vi "LCD Retarder (No Objects).vi"(8 "error in":errorcluster) -> (0 "errorOUT":errorcluster, 3 "LCD out":T1)   [LabVIEW 2015]
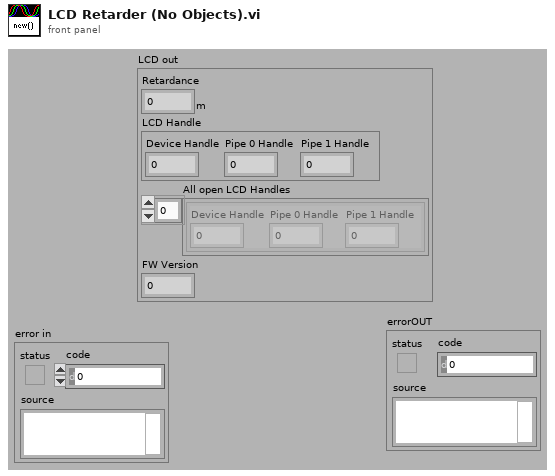
[diagram p1: front panel]
types:
  T1 = cluster{"Retardance":dbl[unit], "LCD Handle":cluster{"Device Handle":u32, "Pipe 0 Handle":u32, "Pipe 1 Handle":u32}, "All open LCD Handles":cluster{"Device Handle":u32, "Pipe 0 Handle":u32, "Pipe 1 Handle":u32}[], "FW Version":dbl}
  T2 = cluster{"Device Handle":u32, "Pipe 0 Handle":u32, "Pipe 1 Handle":u32}[]
  T3 = cluster{"Device Handle":u32, "Pipe 0 Handle":u32, "Pipe 1 Handle":u32}
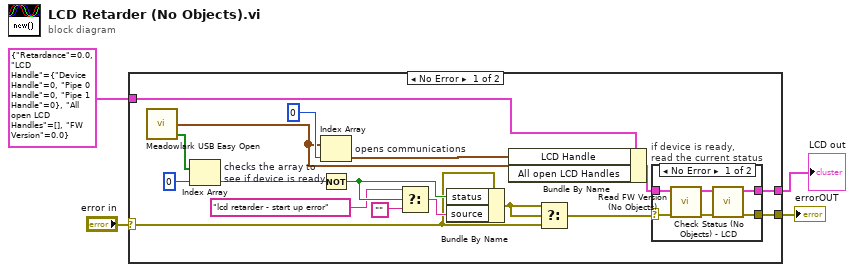
[diagram p0: block diagram]
diagram:
  n1 = case shown="No Error" "error in" {
    selector: "error in" -> [w5 w30]
    tunnel: [w21 w31] -> w2
    tunnel: T1 {"Retardance"=0.0, "LCD Handle"={"Device Handle"=0, "Pipe 0 Handle"=0, "Pipe 1 Handle"=0}, "All open LCD Handles"=[], "FW Version"=0.0} ("Cluster of class private data") -> [w20 w31]
    tunnel: [w18 w30] -> w4
    frame No Error {
      n2 = call "Meadowlark USB Easy Open.vi"() -> ("Device Opened Array"=w13:bool[], "USB Device and Pipes Array"=w8:T2)  [unwired: 1 out]
      n3 = Index Array "checks the array to\nsee if device is ready"(array=w13, index=0) -> (element=w19:bool)
      n4 = Index Array "opens communications"(array=w8, index=0) -> (element=w9:T3)
      n5 = Not(x=w19) -> (.not. x?=w16:bool)
      n6 = Select(t="lcd retarder - start up error", s=w16, f="") -> (s? t:f=w17:string)
      n7 = Bundle By Name(cluster=w5, "status"=w16, "source"=w17) -> (w7:errorcluster)
      n8 = Bundle By Name(cluster=w20, "LCD Handle"=w9, "All open LCD Handles"=w8) -> (w10:T1)
      n9 = Select(t=w7, s=w7, f=w5) -> (s? t:f=w6:errorcluster)
      n10 = case "if device is ready,\nread the current status" shown="No Error" w6 {
        selector: w6 -> [w26 w29]
        tunnel: [w23 w29] -> w18
        tunnel: w10 -> [w27 w28]
        tunnel: [w25 w28] -> w21
        frame No Error {
          n11 = call "Read FW Version (No Objects).vi"("errorIN"=w26, "LCD in"=w27) -> ("error out"=w24:errorcluster, "LCD out"=w22:T1)  [unwired: 7 in, 1 out]
          n12 = call "Check Status (No Objects) - LCD.vi"("error in (no error)"=w24, "Cluster In"=w22) -> ("error out"=w23:errorcluster, "Cluster Out"=w25:T1)  [unwired: 6 in, 2 out]
        }
        frame Error {
        }
      }
    }
    frame Error {
    }
  }
  "errorOUT" <- w4
  "LCD out" <- w2
